vi "Main.vi"(11 "Module Admin":refnum<class "Delacor_lib_QMH_Module Admin.lvclass">) -> ()   [LabVIEW 2020, in "Module.lvlib"]
doc: "This template is based off of the Queued Message Handler design pattern and the Queued Message Handler project template that ships with LabVIEW.\n\nThe main difference is that the queue is private to this module and communication between modules is performed via Broadcast and Request events.\n\nRequest events are wrapped in public API methods and are handled in the Event Handling Loop (EHL) of this VI. Any module can register for Broadcast events sent by this module. The EHL generates messages based on user interface actions.\n\nThe Message Handling Loop (MHL) processes messages generated by the EHL, or by other messages. The messages are string values, so new messages can be added easily to the Message Cases case structure in the MHL. Each message cluster can also provide an optional value for Message Data, which is a variant that can be converted to whatever message-specific data is required.\n_____\nBased on DQMH Project Template 7.0.1.1316."
uses:
  Module.lvlib
  <vilib>/Delacor/Delacor QMH/Libraries/Module Admin_class/Delacor_lib_QMH_Module Admin.lvclass
  Module Data--cluster.ctl
  <vilib>/Delacor/Delacor QMH/Libraries/Message Queue_class/Delacor_lib_QMH_Message Queue.lvclass/Delacor_lib_QMH_Message Queue.ctl
  Stop Argument--cluster.ctl
  <vilib>/Delacor/Delacor QMH/Libraries/Module Admin_class/Delacor_lib_QMH_Module Admin.lvclass/Delacor_lib_QMH_Module Admin.ctl
  <vilib>/Utility/miscctls.llb/LVPointTypeDef.ctl
  <vilib>/Delacor/Delacor QMH/Libraries/Message Queue_class/Delacor_lib_QMH_Enqueue Message (Single).vi
  <vilib>/Delacor/Delacor QMH/Libraries/Module Admin_class/Delacor_lib_QMH_Get External Launch.vi
  <vilib>/Delacor/Delacor QMH/Libraries/Message Queue_class/Delacor_lib_QMH_Message Queue.lvclass
panel:
  out "error out":errorcluster
  out "Status":string
  in  "Simulate MHL Error":bool
  in  "Simulate EHL Error":bool
  # "Other processes communicate with this Module via its Public API (wrappers for its Request Events).\n\nThis Module communicates with other processes via its Broadcast Events.\nAny process that wants to receive these messages can register for this module's Broadcast events."
  # "This template is for the DQMH framework. See the block diagram for more information on how to use this template."
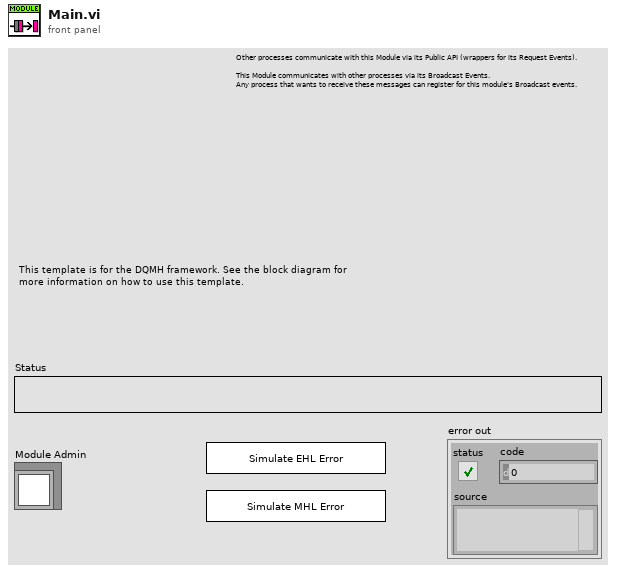
[diagram p1: front panel]
types:
  T1 = typedef "Module.lvlib/Request Events--cluster.ctl" = cluster{"Stop Module":refnum<user-event>, "Show Panel":refnum<user-event>, "Hide Panel":refnum<user-event>, "Get Module Execution Status":refnum<user-event>, "Show Diagram":refnum<user-event>}
  T2 = typedef "Module.lvlib/Module Data--cluster.ctl" = cluster{"Status":string}
  T3 = enum32{"invalid lock state", "Not Locked", "Locked (No Password)", "Password-protected"}
  T4 = typedef "Module.lvlib/Stop Argument--cluster.ctl" = cluster{"Origin":string, "Exit via Stop Module Req?":bool, "Wait for Module to stop?":bool}
  T5 = typedef "LVPointTypeDef.ctl" = cluster{"Horizontal":i16, "Vertical":i16}
  T6 = enum32{"Invalid", "Standard", "Closed", "Hidden", "Minimized", "Maximized"}
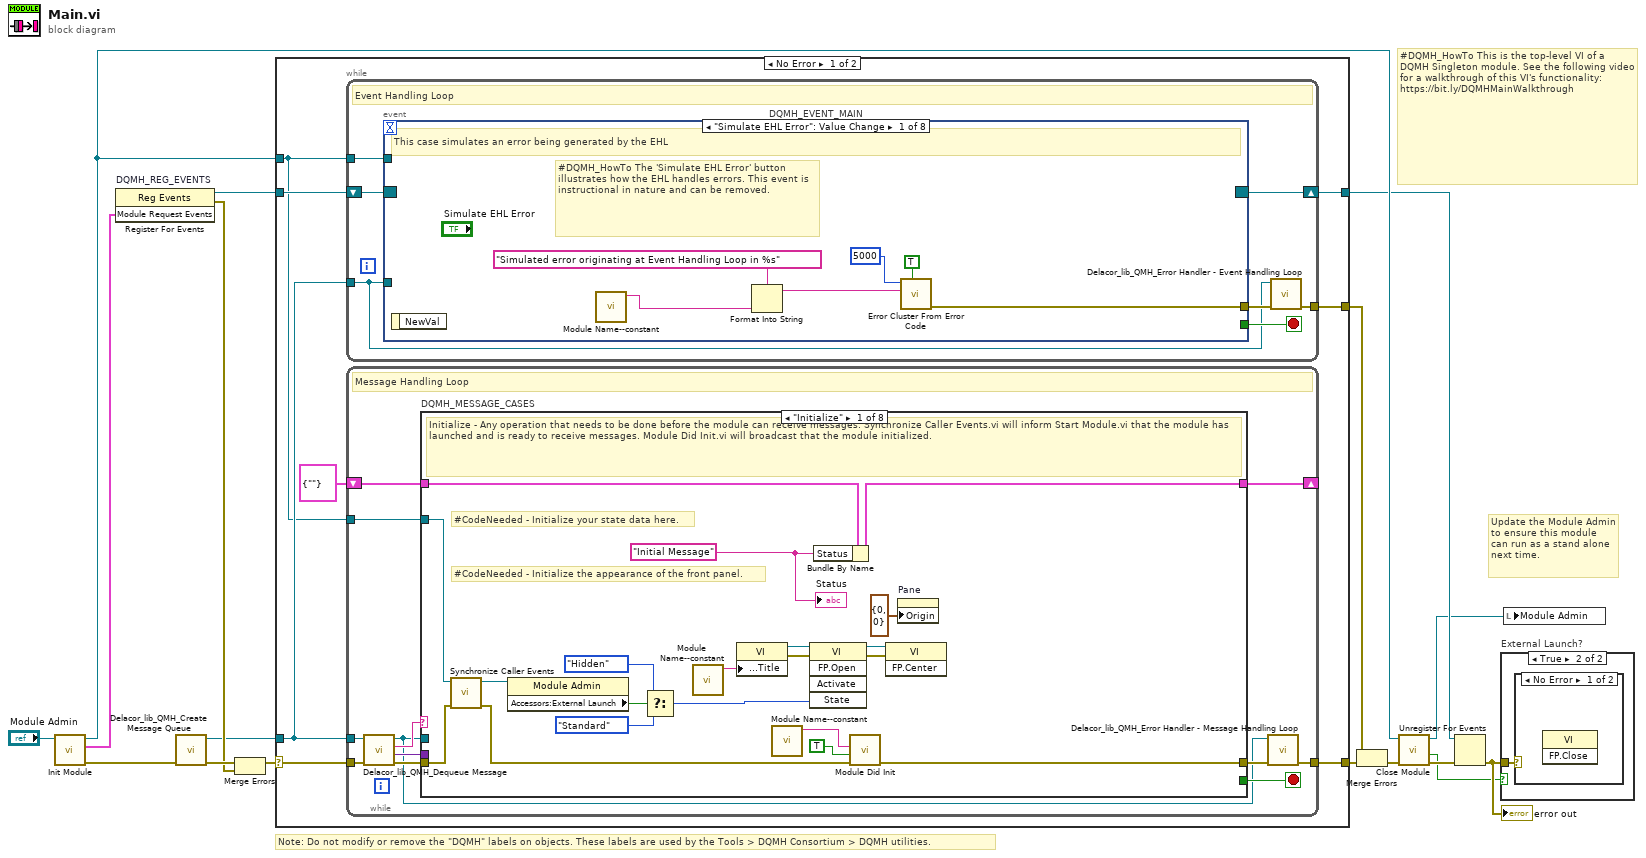
[diagram p0: block diagram]
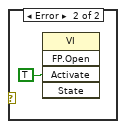
[diagram p3: hidden frame]
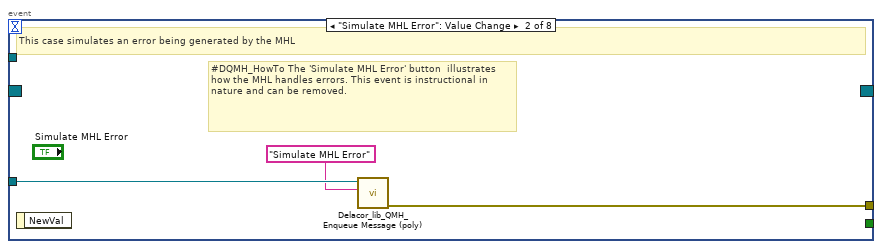
[diagram p4: hidden frame]
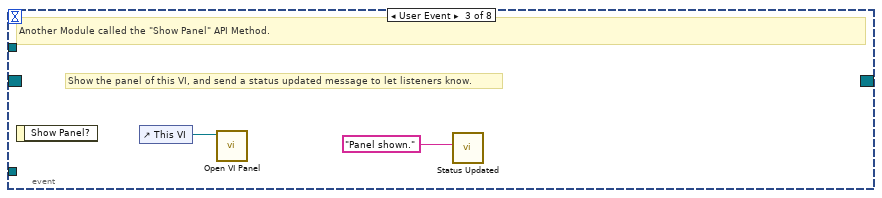
[diagram p5: hidden frame]
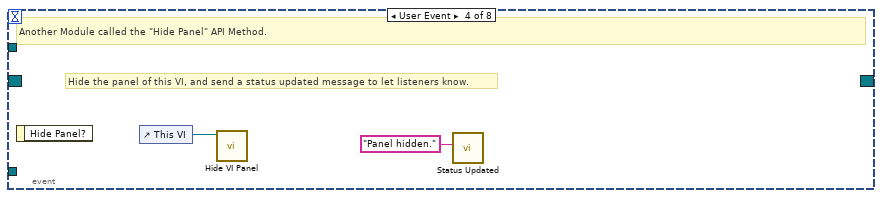
[diagram p6: hidden frame]
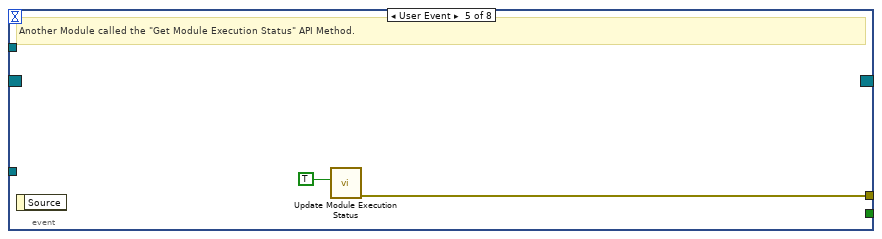
[diagram p7: hidden frame]
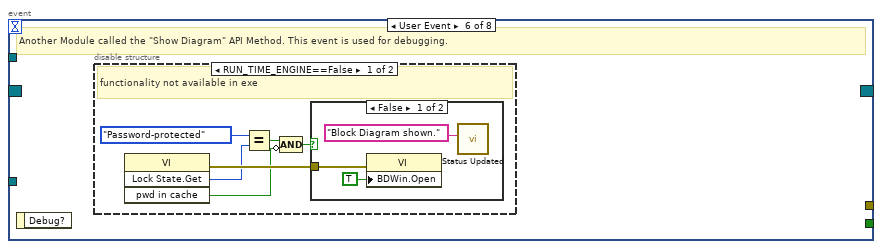
[diagram p8: hidden frame]
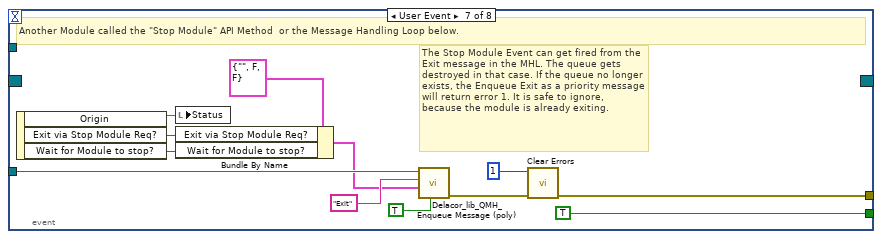
[diagram p11: hidden frame]
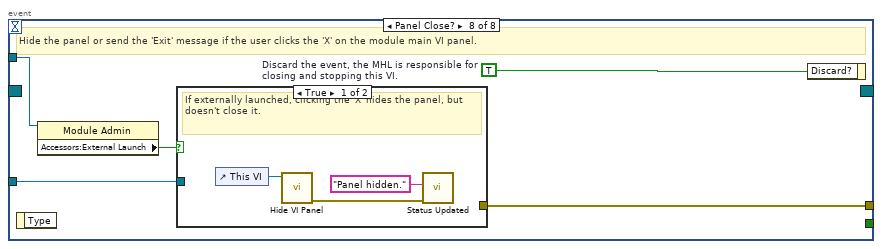
[diagram p12: hidden frame]
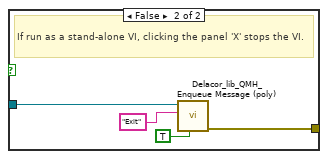
[diagram p13: hidden frame]
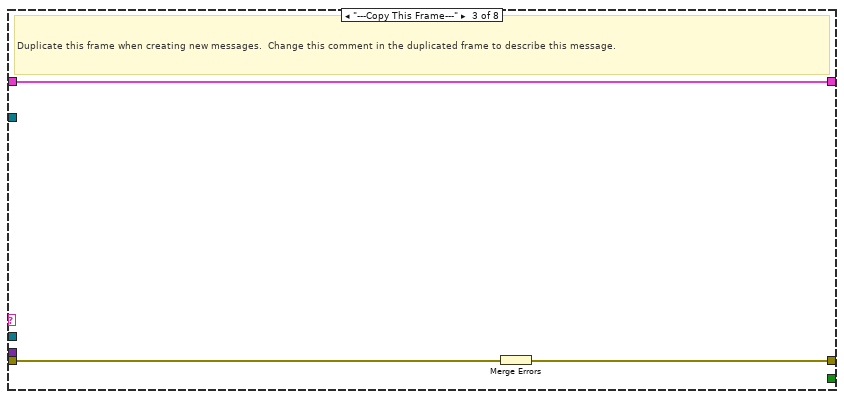
[diagram p15: hidden frame]
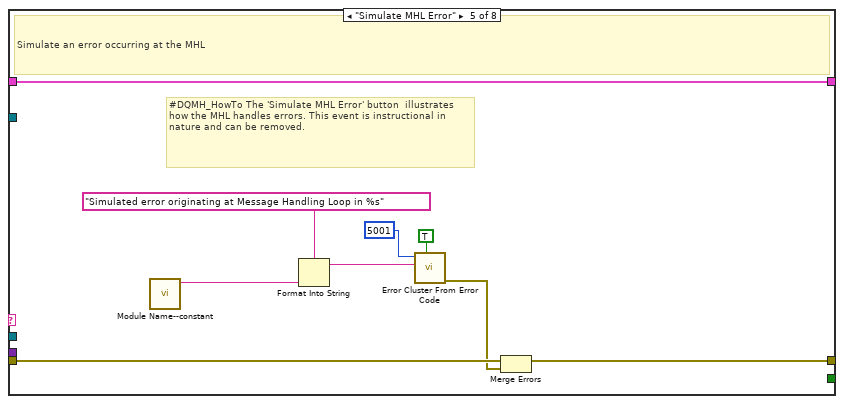
[diagram p17: hidden frame]
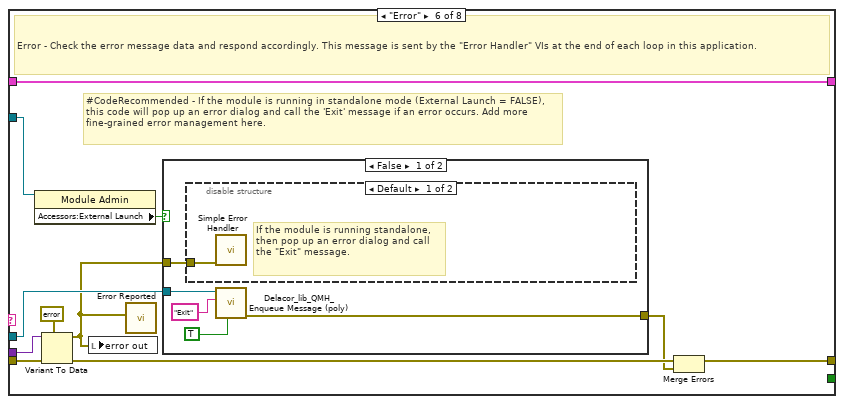
[diagram p18: hidden frame]
diagram:
  # "#DQMH_HowTo This is the top-level VI of a DQMH Singleton module. See the following video for a walkthrough of this VI's functionality: https://bit.ly/DQMHMainWalkthrough"
  # "Note: Do not modify or remove the \"DQMH\" labels on objects. These labels are used by the Tools > DQMH Consortium > DQMH utilities."
  # "Update the Module Admin to ensure this module can run as a stand alone next time."
  n1 = call "Init Module.vi"("Singleton Module Admin in"="Module Admin") -> ("error out"=w16:errorcluster, "Module Request Events"=w5:T1, "Singleton Module Admin out"=w8:refnum<class "Delacor_lib_QMH_Module Admin.lvclass">)  [unwired: 8 in]
  n2 = register-events "DQMH_REG_EVENTS"(w5) -> (reference out=w6:refnum<event-registration>, error out=w9:errorcluster)  [unwired: 2 in]
  n3 = call <vilib>:"Delacor_lib_QMH_Create Message Queue.vi"("error in"=w16) -> ("error out"=w11:errorcluster, "Message Queue"=w4:refnum<class "Delacor_lib_QMH_Message Queue.lvclass">)  [unwired: 9 in]
  n4 = Merge Errors(w11, w9) -> (w10:errorcluster)
  n5 = case shown="No Error" w10 {
    selector: w10 -> [w23 w178]
    tunnel: [w25 w177] -> w17
    tunnel: [w22 w176] -> w7
    tunnel: w6 -> [w20 w176]
    tunnel: w4 -> [w19 w171]
    tunnel: [w24 _] -> w14
    tunnel: w8 -> [w18 w172]
    frame No Error {
      n6 = while {
        tunnel: w19 -> [w26]
        shift-right: [w29] -> w22
        shift-left: w20 -> [w30]
        tunnel: [w31] -> w24
        tunnel: w18 -> [w27]
        stop <- w28 stop-if-true
        # "Event Handling Loop"
        n7 = event "DQMH_EVENT_MAIN" shown="[0] \"Simulate EHL Error\": Value Change" {
          selector: w30 -> [_ _ _ _ _ _ _ _]
          dyn-events: [_ _ _ _ _ _ _ _] -> w29
          timeout: _ -> [_ _ _ _ _ _ _ _]
          tunnel: [_ _ _ _ _ _ TRUE ("Discard?") _] -> w28
          tunnel: w26 -> [_ w40 _ _ _ _ w64 w71]
          tunnel: [w38 w41 _ _ w47 _ w67 w73] -> w32
          tunnel: w27 -> [_ _ _ _ _ _ _ w70]
          event "Simulate EHL Error": Value Change {
            # "#DQMH_HowTo The 'Simulate EHL Error' button  illustrates how the EHL handles errors. This event is instructional in nature and can be removed."
            # "This case simulates an error being generated by the EHL"
            n8 = event-data() -> ()  [unwired: 1 in, 1 out]
            n9 = call "Module Name--constant.vi"() -> ("Module Name"=w35:string)  [unwired: 11 in]
            n10 = Format Into String(format string="Simulated error originating at Event Handling Loop in %s", w35) -> (resulting string=w36:string)  [unwired: 2 in, 1 out]
            n11 = call <vilib>:"Error Cluster From Error Code.vi"("show call chain? (False)"=TRUE, "error message (\"\")"=w36, "error code (0)"=5000) -> ("error out"=w38:errorcluster)  [unwired: 6 in]
          }
          event "Simulate MHL Error": Value Change {
            # "#DQMH_HowTo The 'Simulate MHL Error' button  illustrates how the MHL handles errors. This event is instructional in nature and can be removed."
            # "This case simulates an error being generated by the MHL"
            n12 = event-data() -> ()  [unwired: 1 in, 1 out]
            n13 = call-poly <vilib>:"Delacor_lib_QMH_Enqueue Message (poly).vi"("Message"="Simulate MHL Error", "Message Queue in"=w40) -> ("error out"=w41:errorcluster)  [unwired: 8 in, 1 out]
          }
          event User Event {
            # "Show the panel of this VI, and send a status updated message to let listeners know."
            # "Another Module called the \"Show Panel\" API Method."
            n14 = event-data() -> ()  [unwired: 1 in, 1 out]
            n15 = control-ref of="This VI"() -> (w43:refnum<vi>)
            n16 = call "Open VI Panel.vi"("VI"=w43) -> ()  [unwired: 10 in, 1 out]
            n17 = call "Status Updated.vi"("Status"="Panel shown." ("format string")) -> ()  [unwired: 10 in, 1 out]
          }
          event User Event {
            # "Hide the panel of this VI, and send a status updated message to let listeners know."
            # "Another Module called the \"Hide Panel\" API Method."
            n18 = event-data() -> ()  [unwired: 1 in, 1 out]
            n19 = control-ref of="This VI"() -> (w45:refnum<vi>)
            n20 = call "Hide VI Panel.vi"("VI"=w45) -> ()  [unwired: 10 in, 1 out]
            n21 = call "Status Updated.vi"("Status"="Panel hidden." ("format string")) -> ()  [unwired: 10 in, 1 out]
          }
          event User Event {
            # "Another Module called the \"Get Module Execution Status\" API Method."
            n22 = event-data() -> ()  [unwired: 1 in, 1 out]
            n23 = call "Update Module Execution Status.vi"("Running?"=TRUE) -> ("error out"=w47:errorcluster)  [unwired: 10 in]
          }
          event User Event {
            # "Another Module called the \"Show Diagram\" API Method. This event is used for debugging."
            n24 = event-data() -> ()  [unwired: 1 in, 1 out]
            n25 = disable-structure shown="RUN_TIME_ENGINE==False" {
              frame condition #0 (active) {
                # "functionality not available in exe"
                n26 = invoke on="Invoke Node" class="VI" method="Lock State.Get"() -> (error out=w53:errorcluster, "Get Lock State"=w52:T3, "pwd in cache"=w49:bool)  [unwired: 4 in, 1 out]
                n27 = Equal?(x=T3."Password-protected", y=w52) -> (x = y?=w50:bool)
                n28 = Compound Arithmetic op=AND(w50, invert w49) -> (w48:bool)
                n29 = case shown="False" w48 {
                  tunnel: w53 -> [w56 _]
                  frame False {
                    n30 = property on="Property Node" class="VI"(error in=w56, "BDWin.Open"=TRUE ("Block Diagram Window:Open")) -> ()  [unwired: 1 in, 2 out]
                    n31 = call "Status Updated.vi"("Status"="Block Diagram shown." ("format string")) -> ()  [unwired: 10 in, 1 out]
                  }
                  frame True {
                    # "Password-protected VI, and the password is not in the cache. Do not show the diagram."
                  }
                }
              }
              frame condition #1 {
              }
            }
          }
          event User Event {
            # "The Stop Module Event can get fired from the Exit message in the MHL. The queue gets destroyed in that case. If the queue no longer exists, the Enqueue Exit as a priority message will return error 1. It is safe to ignore, because the module is already exiting."
            # "Another Module called the \"Stop Module\" API Method  or the Message Handling Loop below."
            n32 = event-data() -> ("Origin"=w63:string, "Exit via Stop Module Req?"=w59:bool, "Wait for Module to stop?"=w58:bool)  [unwired: 1 in]
            n33 = local write "Status"(w63) -> ()
            n34 = Bundle By Name(cluster=T4 {"Origin"="", "Exit via Stop Module Req?"=FALSE, "Wait for Module to stop?"=FALSE} ("Stop Argument"), "Exit via Stop Module Req?"=w59, "Wait for Module to stop?"=w58) -> (w57:T4)
            n35 = call-poly <vilib>:"Delacor_lib_QMH_Enqueue Message (poly).vi"("Priority Message? (F)"=TRUE, "Message Data"=w57, "Message"="Exit", "Message Queue in"=w64) -> ("error out"=w68:errorcluster)  [unwired: 6 in, 1 out]
            n36 = call <vilib>:"Clear Errors.vi"("error in (no error)"=w68, "specific error code to clear (0: all)"=1) -> ("error out"=w67:errorcluster)  [unwired: 4 in, 1 out]
          }
          event Panel Close? {
            w72 = TRUE  # Discard the event, the MHL is responsible for closing and stopping this VI.
            # "Hide the panel or send the 'Exit' message if the user clicks the 'X' on the module main VI panel."
            n37 = event-data() -> ()  [unwired: 1 in, 1 out]
            n38 = property on="Property Node" class="Module Admin"(reference=w70) -> ("Accessors:External Launch"=w69:bool)  [unwired: 1 in, 2 out]
            n39 = case shown="True" w69 {
              tunnel: w71 -> [_ w79]
              tunnel: [_ w80] -> w73
              frame True {
                # "If externally launched, clicking the 'X' hides the panel, but doesn't close it."
                n40 = control-ref of="This VI"() -> (w76:refnum<vi>)
                n41 = call "Hide VI Panel.vi"("VI"=w76) -> ("error out"=w74:errorcluster)  [unwired: 10 in]
                n42 = call "Status Updated.vi"("error in"=w74, "Status"="Panel hidden." ("format string")) -> ()  [unwired: 9 in, 1 out]
              }
              frame False {
                # "If run as a stand-alone VI, clicking the panel 'X' stops the VI."
                n43 = call-poly <vilib>:"Delacor_lib_QMH_Enqueue Message (poly).vi"("Priority Message? (F)"=TRUE, "Message"="Exit", "Message Queue in"=w79) -> ("error out"=w80:errorcluster)  [unwired: 7 in, 1 out]
              }
            }
            n44 = event-data ("Event Filter Node")("Discard?"=w72) -> ()  [unwired: 1 in, 1 out]
          }
        }
        n45 = call-dynamic "Delacor_lib_QMH_Error Handler - Event Handling Loop.vi"("error in"=w32, "Message Queue in"=w26) -> ("dup error in"=w31:errorcluster)  [unwired: 8 in, 1 out]
      }
      n46 = while {
        tunnel: w19 -> [w81]
        shift-right: [w89] -> _
        shift-left: T2 {"Status"=""} ("Data Cluster") -> [w90]
        tunnel: w23 -> [w92]
        tunnel: [w84] -> w25
        tunnel: w18 -> [w85]
        stop <- w88 stop-if-true
        # "Message Handling Loop"
        n47 = call-dynamic "Delacor_lib_QMH_Dequeue Message.vi"("error in"=w92, "Message Queue in"=w81) -> ("error out"=w91:errorcluster, "Message Data"=w86:variant, "Message"=w87:string, "Message Queue out"=w82:refnum<class "Delacor_lib_QMH_Message Queue.lvclass">)  [unwired: 6 in]
        n48 = case "DQMH_MESSAGE_CASES" shown="\"Initialize\"" w87 {
          selector: w87 -> [_ _ _ _ _ _ _ w166]
          tunnel: w82 -> [_ _ _ _ _ w132 w154 _]
          tunnel: w91 -> [w110 w114 w117 w119 w128 w139 w160 w169]
          tunnel: [w108 w114 w116 w119 w127 w135 w155 w170] -> w83
          tunnel: w90 -> [w99 w113 w115 w118 w125 w134 w153 w167]
          tunnel: [w98 w113 w115 w118 w125 w134 w153 w167] -> w89
          tunnel: [_ _ _ _ _ _ w152 _] -> w88
          tunnel: w86 -> [_ _ _ _ _ w133 w151 _]
          tunnel: w85 -> [w100 _ _ _ _ w131 w146 _]
          frame "Initialize" {
            w94 = "Initial Message" ("Initial Message")
            # "#CodeNeeded - Initialize the appearance of the front panel."
            # "#CodeNeeded - Initialize your state data here."
            # "Initialize - Any operation that needs to be done before the module can receive messages. Synchronize Caller Events.vi will inform Start Module.vi that the module has launched and is ready to receive messages. Module Did Init.vi will broadcast that the module initialized."
            n49 = call "Synchronize Caller Events.vi"("error in"=w110, "Singleton Module Admin in"=w100) -> ("error out"=w109:errorcluster, "Singleton Module Admin out"=w95:refnum<class "Delacor_lib_QMH_Module Admin.lvclass">)  [unwired: 8 in]
            n50 = property on="Property Node" class="Module Admin"(reference=w95) -> ("Accessors:External Launch"=w104:bool)  [unwired: 1 in, 2 out]
            n51 = Select(t=T6."Hidden" ("State"), s=w104, f=T6."Standard" ("State")) -> (s? t:f=w101:T6)
            n52 = call "Module Name--constant.vi"() -> ("Module Name"=w107:string)  [unwired: 11 in]
            n53 = property on="Property Node" class="VI"("Front Panel.Title"=w107) -> (reference out=w106:refnum<vi>, error out=w112:errorcluster)  [unwired: 2 in]
            n54 = call "Module Name--constant.vi"() -> ("Module Name"=w96:string)  [unwired: 11 in]
            n55 = invoke on="Invoke Node" class="VI" method="FP.Open"(reference=w106, error in=w112, "State"=w101) -> (reference out=w105:refnum<vi>, error out=w111:errorcluster)  [unwired: 2 in, 3 out]
            n56 = Bundle By Name(cluster=w99, "Status"=w94) -> (w98:T2)
            n57 = call "Module Did Init.vi"("error in"=w109, "Initialized?"=TRUE, "Origin"=w96) -> ("error out"=w108:errorcluster)  [unwired: 8 in]
            n58 = invoke on="Invoke Node" class="VI" method="FP.Center"(reference=w105, error in=w111) -> ()  [unwired: 1 in, 3 out]
            n59 = property on="Pane" class="Pane"("Origin"=T5 {"Horizontal"=0, "Vertical"=0}) -> ()  [unwired: 2 in, 2 out]
            "Status" <- w94
          }
          frame "---Module Specific---" {
            # "Separator -- The following cases handle messages specific to this Module."
          }
          frame "---Copy This Frame---" {
            # "Duplicate this frame when creating new messages.  Change this comment in the duplicated frame to describe this message."
            n60 = Merge Errors(w117) -> (w116:errorcluster)
          }
          frame "---Exit and Error Handling---" {
            # "Separator - The following cases handle errors and exit messages."
          }
          frame "Simulate MHL Error" {
            # "#DQMH_HowTo The 'Simulate MHL Error' button  illustrates how the MHL handles errors. This event is instructional in nature and can be removed."
            # "Simulate an error occurring at the MHL"
            n61 = call "Module Name--constant.vi"() -> ("Module Name"=w121:string)  [unwired: 11 in]
            n62 = Format Into String(format string="Simulated error originating at Message Handling Loop in %s", w121) -> (resulting string=w122:string)  [unwired: 2 in, 1 out]
            n63 = call <vilib>:"Error Cluster From Error Code.vi"("show call chain? (False)"=TRUE, "error message (\"\")"=w122, "error code (0)"=5001) -> ("error out"=w126:errorcluster)  [unwired: 6 in]
            n64 = Merge Errors(w128, w126) -> (w127:errorcluster)
          }
          frame "Error" {
            # "#CodeRecommended - If the module is running in standalone mode (External Launch = FALSE), this code will pop up an error dialog and call the 'Exit' message if an error occurs. Add more fine-grained error management here."
            # "Error - Check the error message data and respond accordingly. This message is sent by the \"Error Handler\" VIs at the end of each loop in this application."
            n65 = property on="Property Node" class="Module Admin"(reference=w131) -> ("Accessors:External Launch"=w130:bool)  [unwired: 1 in, 2 out]
            n66 = Variant To Data(error in=w139, type=errorcluster {"status"=FALSE, "code"=0, "source"=""} ("error constant"), Variant=w133) -> (data=w129:errorcluster, error out=w137:errorcluster)
            n67 = local write "error out"(w129) -> ()
            n68 = call "Error Reported.vi"("Error"=w129) -> ()  [unwired: 10 in, 1 out]
            n69 = case shown="False" w130 {
              tunnel: [w144 _] -> w136
              tunnel: w132 -> [w142 _]
              tunnel: w129 -> [w143 _]
              frame False {
                n70 = disable-structure shown="Default" {
                  disable-tunnel: w143 -> [w145 _]
                  frame condition #0 (active) {
                    # "If the module is running standalone, then pop up an error dialog and call the \"Exit\" message."
                    n71 = call <vilib>:"Simple Error Handler.vi"("error in (no error)"=w145) -> ()  [unwired: 4 in, 5 out]
                  }
                  frame condition #1 {
                    # "To prevent the Simple Error Handler VI from being loaded (e.g. when deploying to a Real-Time target), add the Conditional Disable Symbol \"DQMH_Disable_SEH\" to your project and set it to TRUE."
                  }
                }
                n72 = call-poly <vilib>:"Delacor_lib_QMH_Enqueue Message (poly).vi"("Priority Message? (F)"=TRUE, "Message"="Exit", "Message Queue in"=w142) -> ("error out"=w144:errorcluster)  [unwired: 7 in, 1 out]
              }
              frame True {
                # "If the module was launched externally, calling the Error Reported broadcast VI is the only action performed by the \"Error\" message. The module's caller can then process the error appropriately."
              }
            }
            n73 = Merge Errors(w137, w136) -> (w135:errorcluster)
          }
          frame "Exit" {
            w150 = 91  # 91: not all Exit messages will have an argument
            w152 = TRUE  # Stop the VI
            # "Release the message queue reference"
            # "#CodeNeeded - Add any required cleanup code here."
            # "Exit - Exit the application."
            n74 = Variant To Data(error in=w160, type=T4 {"Origin"="", "Exit via Stop Module Req?"=FALSE, "Wait for Module to stop?"=FALSE} ("Stop Argument"), Variant=w151) -> (data=w148:T4, error out=w157:errorcluster)
            n75 = call <vilib>:"Clear Errors.vi"("error in (no error)"=w157, "specific error code to clear (0: all)"=w150) -> ("error out"=w159:errorcluster)  [unwired: 4 in, 1 out]
            n76 = control-ref of="This VI"() -> (w147:refnum<vi>)
            n77 = call-dynamic "Delacor_lib_QMH_Release Message Queue.vi"("error in"=w159, "Message Queue"=w154) -> ("error out"=w158:errorcluster)  [unwired: 9 in]
            n78 = call "Handle Exit.vi"("Stop Argument"=w148, "Admin in"=w146, "VI reference"=w147) -> ("error out"=w156:errorcluster)  [unwired: 7 in, 1 out]
            n79 = Merge Errors(w158, w156) -> (w155:errorcluster)
            n80 = call "Error Reported.vi"("Error"=w155) -> ()  [unwired: 10 in, 1 out]
          }
          frame Default {
            # "'Default' case only runs if there is a message that isn't defined in any of the other cases.  Output a programming error."
            n81 = call "Module Name--constant.vi"() -> ("Module Name"=w165:string)  [unwired: 11 in]
            n82 = Format Into String(format string="The invalid message string \"%s\" was received in the Message Handling Loop for module \"%s\".", w166, w165) -> (resulting string=w161:string)  [unwired: 2 in, 1 out]
            n83 = call <vilib>:"Error Cluster From Error Code.vi"("show call chain? (False)"=TRUE, "error message (\"\")"=w161, "error code (0)"=1) -> ("error out"=w168:errorcluster)  [unwired: 6 in]
            n84 = Merge Errors(w169, w168) -> (w170:errorcluster)
          }
        }
        n85 = call-dynamic "Delacor_lib_QMH_Error Handler - Message Handling Loop.vi"("error in"=w83, "Message Queue in"=w82) -> ("dup error in"=w84:errorcluster)  [unwired: 8 in, 1 out]
      }
    }
    frame Error {
      # "Synchronize Caller Events.vi will inform Start Module.vi that the module has launched and will let the code calling Start Module.vi register for broadcasts and would permit the caller receive the broadcast that an error occurred at launch time."
      n86 = call-dynamic "Delacor_lib_QMH_Release Message Queue.vi"("error in"=w178, "Message Queue"=w171) -> ("error out"=w177:errorcluster)  [unwired: 9 in]
      n87 = call "Synchronize Caller Events.vi"("Singleton Module Admin in"=w172) -> ("error out"=w179:errorcluster)  [unwired: 9 in, 1 out]
      n88 = call "Module Name--constant.vi"() -> ("Module Name"=w175:string)  [unwired: 11 in]
      n89 = Format Into String(format string="An error occurred during initialization. %s is no longer running.", w175) -> (resulting string=w173:string)  [unwired: 2 in, 1 out]
      n90 = Merge Errors(w177, w179) -> (w180:errorcluster)
      n91 = call "Error Reported.vi"("Additional Information"=w173, "Error"=w180) -> ()  [unwired: 9 in, 1 out]
    }
  }
  n92 = Merge Errors(w14, w17) -> (w13:errorcluster)
  n93 = call "Close Module.vi"("error in"=w13, "Module Admin in"=w8) -> ("error out"=w15:errorcluster, "External Launch"=w1:bool, "Module Admin out"=w2:refnum<class "Delacor_lib_QMH_Module Admin.lvclass">)  [unwired: 7 in]
  n94 = Unregister For Events(event registration refnum=w7, error in=w15) -> (error out=w12:errorcluster)
  "error out" <- w12
  n95 = case "External Launch?" shown="True" w1 {
    tunnel: w12 -> [_ w181]
    frame False {
    }
    frame True {
      n96 = case shown="No Error" w181 {
        frame No Error {
          n97 = invoke on="Invoke Node" class="VI" method="FP.Close"() -> ()  [unwired: 3 in, 3 out]
        }
        frame Error {
          n98 = invoke on="Invoke Node" class="VI" method="FP.Open"("Activate"=TRUE ("Activate?")) -> ()  [unwired: 4 in, 5 out]
        }
      }
    }
  }
  n99 = local write "Module Admin"(w2) -> ()
